vi "Write A.vi"(8 "error in (no error)":errorcluster, 10 "A":dbl, 11 "Arithmetic Operations in":refnum<class "Arithmetic Operations.lvclass">) -> (0 "error out":errorcluster, 3 "Arithmetic Operations out":refnum<class "Arithmetic Operations.lvclass">)   [LabVIEW 2020, in "Arithmetic Operations.lvclass"]
uses:
  Arithmetic Operations.lvclass
  Arithmetic Operations.lvclass/Arithmetic Operations.ctl
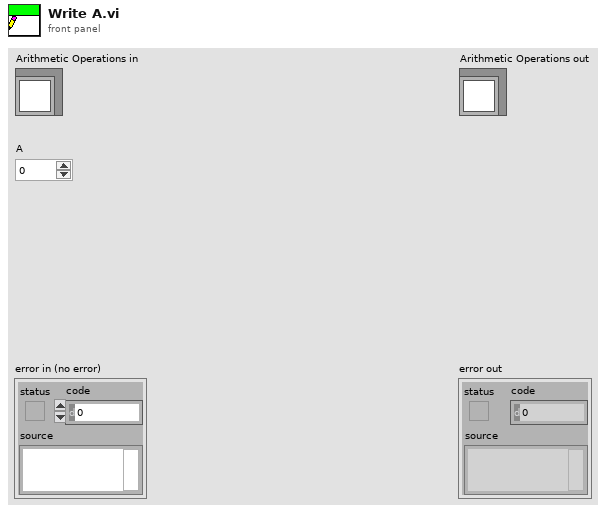
[diagram p1: front panel]
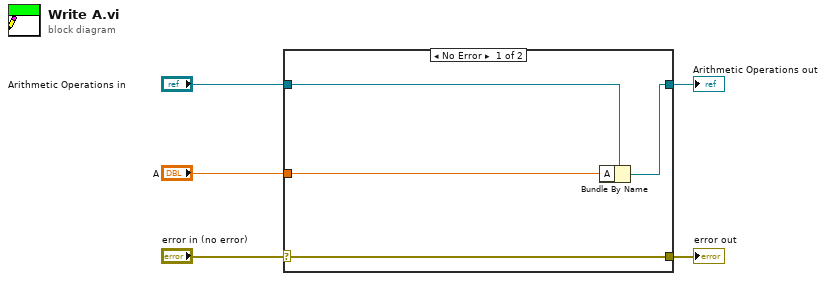
[diagram p0: block diagram]
diagram:
  n1 = case shown="No Error" "error in (no error)" {
    selector: "error in (no error)" -> [w9 w10]
    tunnel: [w9 w10] -> w4
    tunnel: [w7 w11] -> w2
    tunnel: "Arithmetic Operations in" -> [w8 w11]
    tunnel: "A" -> [w6 _]
    frame No Error {
      n2 = Bundle By Name(cluster=w8, "A"=w6) -> (w7:refnum<class "Arithmetic Operations.lvclass">)
    }
    frame Error {
    }
  }
  "error out" <- w4
  "Arithmetic Operations out" <- w2
